vi "GetMCListboxIndex.vi"(8 "error in (no error)":errorcluster, 11 "Control in":refnum<vi>) -> (0 "error out":errorcluster, 1 "Size":i32, 2 "Index":i32, 3 "MCListbox out":refnum<vi>)   [LabVIEW 2020, in "ContextHelpEditor.lvlib"]
uses:
  ContextHelpEditor.lvlib
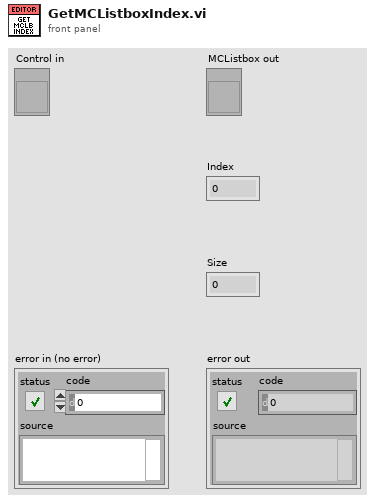
[diagram p1: front panel]
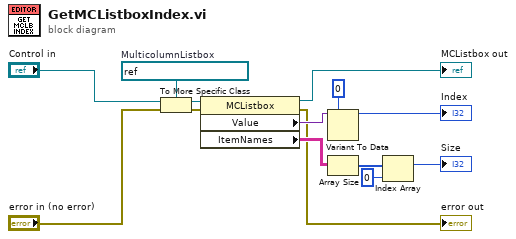
[diagram p0: block diagram]
diagram:
  w14 = refnum<vi> refnum  # MulticolumnListbox
  n1 = To More Specific Class(target class=w14, reference="Control in", error in="error in (no error)") -> (specific class reference=w11:refnum<vi>, error out=w12:errorcluster)
  n2 = property class="MCListbox"(reference=w11, error in=w12) -> (reference out=→"MCListbox out":refnum<vi>, error out=→"error out":errorcluster, "Value"=w6:variant, "ItemNames"=w10:string[][])
  n3 = Variant To Data(type=0 ("index"), Variant=w6) -> (data=→"Index":i32)  [unwired: 1 in, 1 out]
  n4 = Array Size(array=w10) -> (size(s)=w9:i32[])
  n5 = Index Array(array=w9, index=0) -> (element=→"Size":i32)
